vi "TEST - Get Variant Attributes.vi"(8 "error in (no error)":errorcluster) -> (0 "error out":errorcluster, 2 "pass":bool)   [LabVIEW 2020]
uses:
  source/library/Type Descriptor Enumeration.ctl
panel:
  out "Failures":T1(array[cluster])
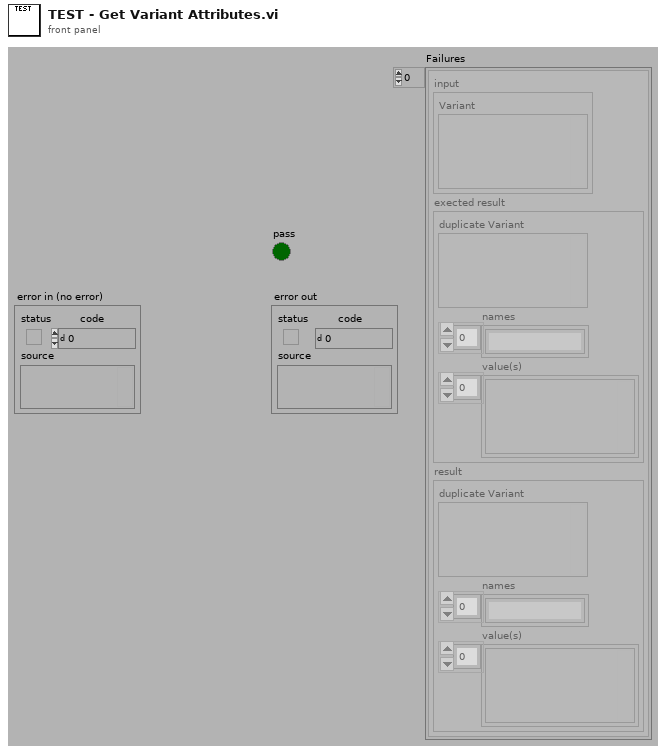
[diagram p1: front panel]
types:
  T1 = cluster{"input":cluster{"Variant":variant}, "exected result":cluster{"duplicate Variant":variant, "names":string[], "value(s)":variant[]}, "result":cluster{"duplicate Variant":variant, "names":string[], "value(s)":variant[]}}[]
  T2 = typedef "Type Descriptor Enumeration.ctl" = enum8{"<Null>", "I8", "I16", "I32", "I64", "U8", "U16", "U32", "U64", "SGL", "DBL", "EXT", "CSG", "CDB", "CXT", "0x0F", "0x10", "0x11", "0x12", "0x13", "0x14", "Enum U8", "Enum U16", "Enum U32", "Enum U64", "SGL PQ", "DBL PQ", "EXT PQ", "CSG PQ", "CDB PQ", "CXT PQ", "0x1F", "0x20", "Boolean", "0x22", "0x23", "0x24", "0x25", "0x26", "0x27", "0x28", "0x29", "0x2A", "0x2B", "0x2C", "0x2D", "0x2E", "0x2F", "String", "0x31", "Path", "Pict", "0x34", "0x35", "0x36", "DAQ", "0x38", "0x39", "0x3A", "0x3B", "0x3C", "0x3D", "0x3E", "0x3F", "Array", "0x41", "0x42", "0x43", "0x44", "0x45", "0x46", "0x47", "0x48", "0x49", "0x4A", "0x4B", "0x4C", "0x4D", "0x4E", "0x4F", "Cluster", "0x51", "0x52", "Variant", "Waveform", "0x55", "0x56", "0x57", "0x58", "0x59", "0x5A", "0x5B", "0x5C", "0x5D", "0x5E", "Fixed Point", "0x60", "0x61", "0x62", "0x63", "0x64", "0x65", "0x66", "0x67", "0x68", "0x69", "0x6A", "0x6B", "0x6C", "0x6D", "0x6E", "0x6F", "Refnum", "0x71", "0x72", "Set Collection", "Map Collection"}
  T3 = cluster{"input":cluster{"Variant":variant}, "exected result":cluster{"duplicate Variant":variant, "names":string[], "value(s)":variant[]}, "result":cluster{"duplicate Variant":variant, "names":string[], "value(s)":variant[]}}
  T4 = cluster{"duplicate Variant":variant, "names":string[], "value(s)":variant[]}
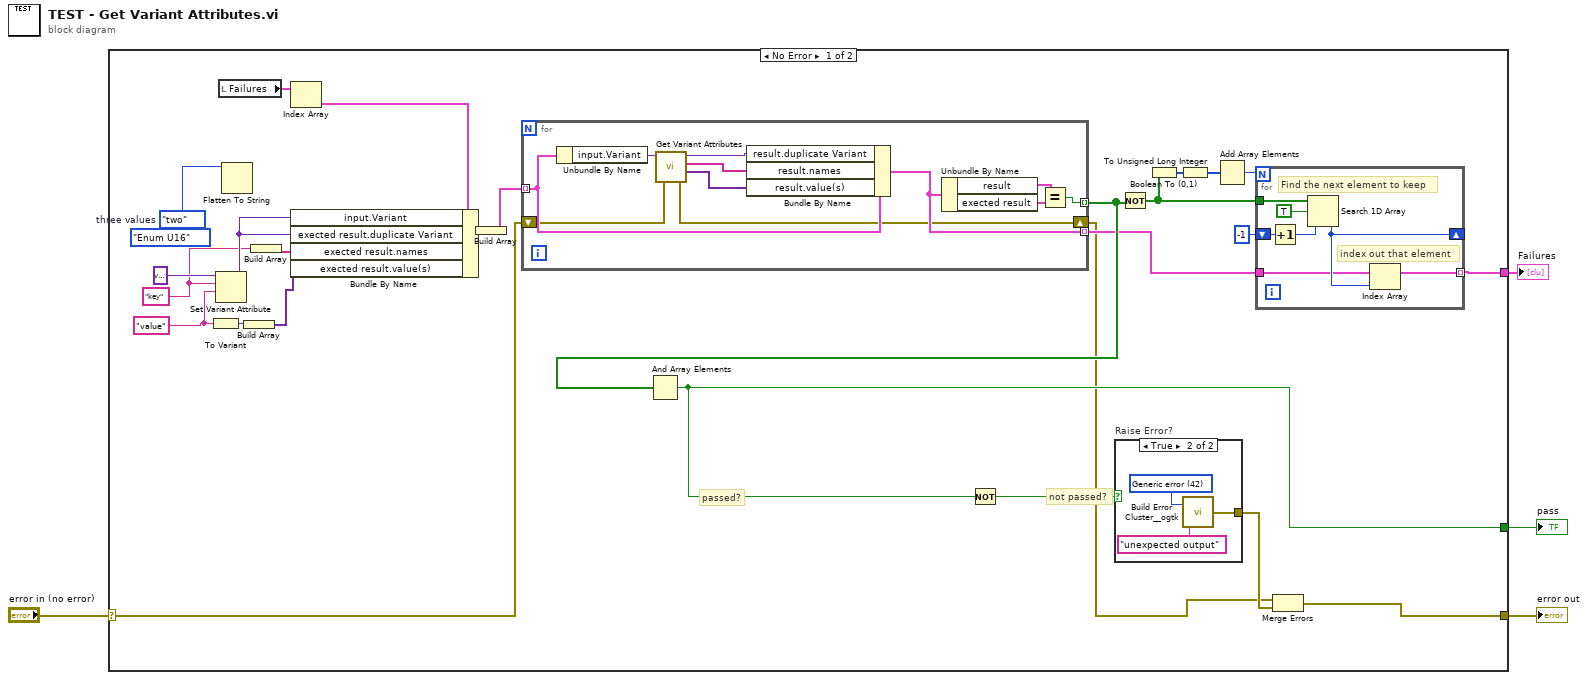
[diagram p0: block diagram]
diagram:
  n1 = case shown="No Error" "error in (no error)" {
    selector: "error in (no error)" -> [w16 w52]
    tunnel: [w27 _] -> w4
    tunnel: [w30 w52] -> w2
    tunnel: [w19 _] -> w1
    frame No Error {
      (unwired) Type_Descriptor_Enumeration."Enum U16" ("exected result.Type Descriptor Enumeration")
      w13 = enum16{"one", "two", "three"}."two"  # three values
      w7 = "value" ("name")
      w8 = "key" ("name")
      # "not passed?"
      # "passed?"
      n2 = To Variant(anything=w7) -> (Variant=w6:variant)
      n3 = Set Variant Attribute(Variant=variant, name=w8, value=w7) -> (Variant out=w10:variant)  [unwired: 1 in, 2 out]
      n4 = local read "Failures"() -> (w14:T1)
      n5 = Flatten To String(anything=w13) -> ()  [unwired: 3 in, 3 out]
      n6 = Build Array(w6) -> (w5:variant[])
      n7 = Build Array(w8) -> (w9:string[])
      n8 = Index Array(array=w14) -> (element=w12:T3)  [unwired: 1 in]
      n9 = Bundle By Name(cluster=w12, "input.Variant"=w10, "exected result.duplicate Variant"=w10, "exected result.names"=w9, "exected result.value(s)"=w5) -> (w18:T3)
      n10 = Build Array(w18) -> (w17:T1)
      n11 = for {
        tunnel: w17 -> [w47] mode=indexing
        tunnel: [w48] -> w21 mode=indexing
        tunnel: [w46] -> w20 mode=indexing
        shift-right: [w42] -> w15
        shift-left: w16 -> [w41]
        n12 = Unbundle By Name(w47) -> ("input.Variant"=w43:variant)
        n13 = call "Get Variant Attributes.vi"("error in"=w41, "Variant"=w43) -> ("error out"=w42:errorcluster, "value(s)"=w38:variant[], "names"=w39:string[], "duplicate Variant"=w40:variant)  [unwired: 2 in]
        n14 = Bundle By Name(cluster=w47, "result.duplicate Variant"=w40, "result.names"=w39, "result.value(s)"=w38) -> (w46:T3)
        n15 = Unbundle By Name(w46) -> ("result"=w45:T4, "exected result"=w44:T4)
        n16 = Equal?(x=w45, y=w44) -> (x = y?=w48:bool)
      }
      n17 = And Array Elements(Boolean array=w21) -> (logical AND=w27:bool)
      n18 = Not(x=w27) -> (.not. x?=w28:bool)
      n19 = case "Raise Error?" shown="True" w28 {
        tunnel: [_ w49] -> w29
        frame False {
        }
        frame True {
          w50 = 42 items=["No error", "Argument error", "Memory is full", "Out of zone", "End of file", "File already open", "Generic file I/O error", "File not found", "File permission error", "Disk is full", "Duplicate path", "Too many files open", "System feature not enabled", "Resource file not found", "Cannot add resource", "Resource not found", "Image not found", "Image memory error", "Pen does not exist", "Config type invalid", "Config token not found", "Config parse error", "Config memory error", "Bad external code format", "Bad external code offset", "External code not present", "Null window", "Destroy window error", "Null menu", "Print aborted", "Bad print record", "Print driver error", "Windows error during printing", "Memory error during printing", "Print dialog error", "Generic print error", "Invalid device refnum", "Device not found", "Device parameter error", "Device unit error", "Cannot open device", "Device call aborted", "Generic error", "Cancelled by user", "Object ID too low", "Object ID too high", "Object not in heap", "Unknown heap", "Unknown object (invalid DefProc)", "Unknown object (DefProc not in table)", "Message out of range", "Invalid (null) method", "Unknown message", "Manager call not supported", "Bad address", "Network operation in progress", "Network operation timed out", "Connection is busy", "Network attribute not supported", "Network error", "Address in use", "System out of memory", "Connection aborted", "Connection refused", "Not connected", "Already connected", "Connection closed", "Initialization error (interapplication manager)", "Bad occurrence", "Wait on unbound occurrence handler", "Occurrence queue overflow", "Datalog type conflict", "Unused", "Unrecognized type (interapplication manager)", "Memory corrupt", "Failed to make temporary DLL", "Old CIN version", "Drag socket not found", "Failed to load drop-object", "Failed to register OLE object", "Failed to release OLE object", "Format specifier type mismatch", "Unknown format specifier", "Too few format specifiers", "Too many format specifiers", "Scan failed", "Newer CIN version", "Error converting to variant", "Runtime menu error", "Password tampered", "Variant attribute not found", "Incompatible variant data type", "Event data is not available", "Event Store is not present", "Occurrence is not found", "Event Queue is not created", "Event info is not available", "Refnum passed is NULL", "Error retrieving Class GUID", "Error retrieving CoClass GUID", "Error retrieving TypeLib GUID.", "Bad built application magic bytes.", "Specific driver is different from the specific driver associated with the Logical Name.", "There is no session opened to the class driver.", "Max Error", "MAX - Error with config objects", "MAX - Error loading configuration", "MAX - Group not supported"]
          n20 = call <userlib>:"Build Error Cluster__ogtk.vi"("String to Prepend to source (\"\")"="unexpected output" ("String to Prepend to source (\"\")"), "code"=w50) -> ("error out"=w49:errorcluster)
        }
      }
      n21 = Not(x=w21) -> (.not. x?=w23:bool[])
      n22 = Boolean To (0,1)(Boolean=w23) -> (0, 1=w24:i16[])
      n23 = To Unsigned Long Integer(number=w24) -> (unsigned 32bit integer=w22:u32[])
      n24 = Add Array Elements(numeric array=w22) -> (sum=w25:u32)
      n25 = for {
        N: w25 -> [_]
        tunnel: w20 -> [w33]
        tunnel: w23 -> [w37]
        shift-right: [w34] -> _
        shift-left: -1 ("start index (0)") -> [w35]
        tunnel: [w32] -> w19 mode=indexing
        # "index out that element"
        # "Find the next element to keep"
        n26 = Increment(x=w35) -> (x+1=w31:i32)
        n27 = Search 1D Array(1D array=w37, element=TRUE, start index (0)=w31) -> (index of element=w34:i32)
        n28 = Index Array(array=w33, index=w34) -> (element=w32:T3)
      }
      n29 = Merge Errors(w15, w29) -> (w30:errorcluster)
    }
    frame Error {
    }
  }
  "pass" <- w4
  "error out" <- w2
  "Failures" <- w1
